vi "TCPHandler.vi"(5 "result Types":variant, 8 "method":string, 9 "params":variant, 11 "connection ID":refnum<k5>) -> (0 "method":string, 1 "result":variant, 3 "connection ID":refnum<k5>)   [LabVIEW 2016]
panel:
  out "JSON-request":string
  out "JSON-response":string
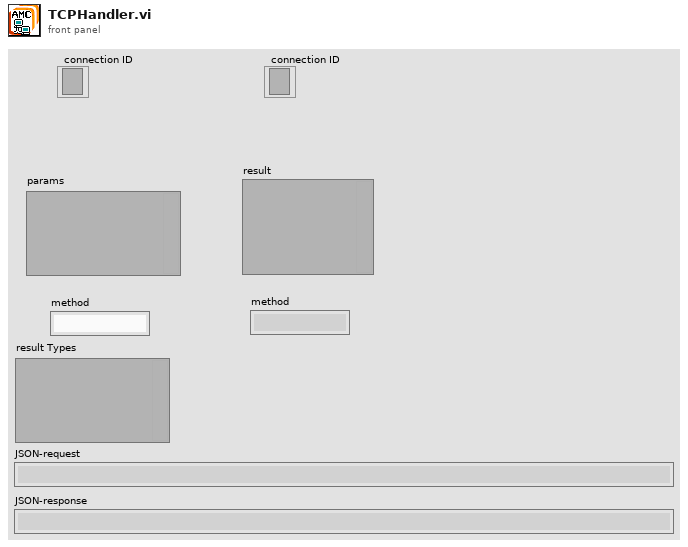
[diagram p1: front panel]
types:
  T1 = enum16{"Standard", "Buffered", "CRLF", "Immediate"}
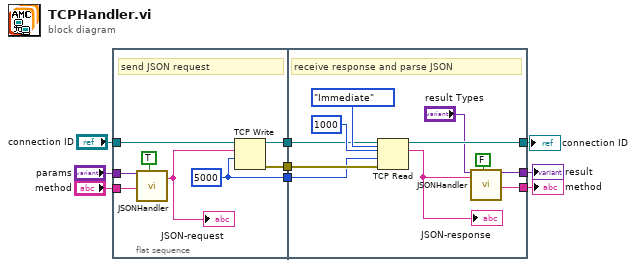
[diagram p0: block diagram]
diagram:
  n1 = flat-sequence {
    tunnel: "connection ID" -> [w17]
    tunnel: "params" -> [w14]
    tunnel: "method" -> [w13]
    tunnel: [w11] -> w4
    tunnel: [w12] -> w3
    tunnel: [w10] -> w1
    tunnel: [w21] -> w5
    tunnel: [w23] -> w8
    tunnel: w4 -> [w25]
    tunnel: w3 -> [w24]
    tunnel: [w22] -> w2
    tunnel: w1 -> [w19]
    frame #0 {
      w10 = 5000 ("timeout ms (25000)")
      # "send JSON request"
      n2 = call "JSONHandler.vi"("params"=w14, "method"=w13, "Set"=TRUE) -> ("JSON-request"=w15:string)  [unwired: 12 in, 4 out]
      "JSON-request" <- w15
      n3 = TCP Write(connection ID=w17, data in=w15, 9:w10) -> (connection ID out=w11:refnum<k5>, error out=w12:errorcluster)  [unwired: 1 in, 1 out]
    }
    frame #1 {
      # "receive response and parse JSON"
      n4 = TCP Read(connection ID=w25, bytes to read=1000, error in (no error)=w24, 7:T1."Immediate" ("mode (standard)"), 9:w19) -> (connection ID out=w23:refnum<k5>, data out=w20:string)  [unwired: 1 out]
      "JSON-response" <- w20
      n5 = call "JSONHandler.vi"("params"="result Types", "JSON-response"=w20, "Set"=FALSE) -> ("result"=w22:variant, "method"=w21:string)  [unwired: 12 in, 3 out]
    }
  }
  "connection ID" <- w8
  "result" <- w2
  "method" <- w5
